vi "Basic Set Cursor.vi"(8 "error in (no error)":errorcluster, 9 "position":cluster{"row":i8, "column":i8}, 11 "cluster of private data":T1={"FPGA VI Reference"=refnum, "device index"=0, "screen size"=enum."8x1", "font size"=enum."5x8", "auto wrap"=FALSE, "alignment"=enum."None", "number of line"=enum."2 lines", "shift 0"=0, "entry mode 0"=enum."increment & no shift", "shift 1"=0, "entry mode 1"=enum."increment & no shift"}) -> (0 "error out":errorcluster, 3 "cluster of private data out":T1={"FPGA VI Reference"=refnum, "device index"=0, "screen size"=enum."8x1", "font size"=enum."5x8", "auto wrap"=FALSE, "alignment"=enum."None", "number of line"=enum."2 lines", "shift 0"=0, "entry mode 0"=enum."increment & no shift", "shift 1"=0, "entry mode 1"=enum."increment & no shift"}, 4 "chip select":enum16{"1st chip", "2nd chip"}(ring))   [LabVIEW 2017, in "HD44780.lvclass"]
uses:
  HD44780.lvclass
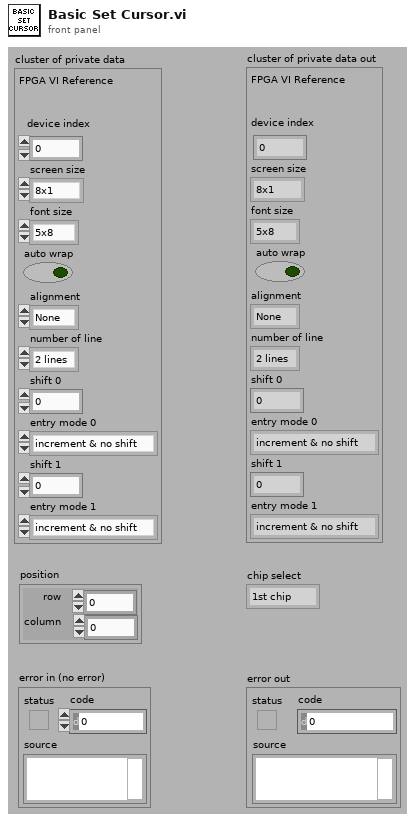
[diagram p1: front panel]
types:
  T1 = cluster{"FPGA VI Reference":refnum<k20>, "device index":i8, "screen size":enum8{"8x1", "8x2", "12x4", "16x1", "16x2", "16x4", "20x1", "20x2", "20x4", "24x1", "24x2", "40x2", "40x4"}, "font size":enum8{"5x8", "5x10"}, "auto wrap":bool, "alignment":enum16{"None", "Left", "Center", "Right"}, "number of line":enum8{"1 line", "2 lines"}, "shift 0":i8, "entry mode 0":enum8{"increment & no shift", "increment & shift", "decrement & no shift", "decrement & shift"}, "shift 1":i8, "entry mode 1":enum8{"increment & no shift", "increment & shift", "decrement & no shift", "decrement & shift"}}
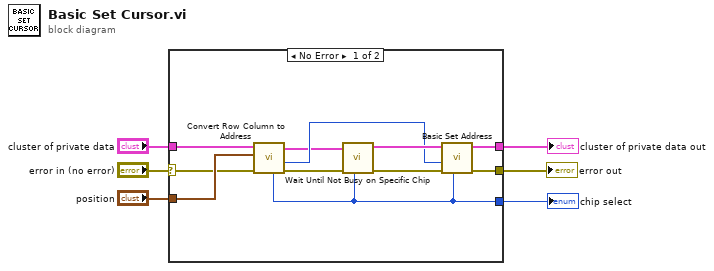
[diagram p0: block diagram]
diagram:
  n1 = case shown="No Error" "error in (no error)" {
    selector: "error in (no error)" -> [w13 w19]
    tunnel: "cluster of private data" -> [w14 w18]
    tunnel: "position" -> [w17 _]
    tunnel: [w16 w19] -> w4
    tunnel: [w15 w18] -> w2
    tunnel: [w9 _] -> w1
    frame No Error {
      n2 = call "Convert Row Column to Address.vi"("error in (no error)"=w13, "cursor position"=w17, "cluster of private data in"=w14) -> ("error out"=w7:errorcluster, "address"=w10:u8, "cluster of private data out"=w8:T1, "chip select"=w9:enum16{"1st chip", "2nd chip"})  [unwired: 5 in]
      n3 = call "Wait Until Not Busy on Specific Chip.vi"("chip select  (1st chip)"=w9, "error in (no error)"=w7, "cluster of private data in"=w8) -> ("error out"=w12:errorcluster, "cluster of private data out"=w11:T1)  [unwired: 7 in]
      n4 = call "Basic Set Address.vi"("chip select  (1st chip)"=w9, "error in (no error)"=w12, "address (0, 0)"=w10, "cluster of private data in"=w11) -> ("error out"=w16:errorcluster, "cluster of private data out"=w15:T1)  [unwired: 6 in]
    }
    frame Error {
    }
  }
  "error out" <- w4
  "cluster of private data out" <- w2
  "chip select" <- w1
